vi "demo02_test.vi"() -> ()   [LabVIEW 2017]
panel:
  out "字符串长度":dbl
  in  "字符串":string
  out "数组":dbl[][](array[numeric])
  out "布尔":bool
  out "次数 2":i32
  out "次数":i32
  out "波形图表":dbl(graph)
  out "数值 6":dbl
  in  "数值 5":dbl
  in  "数值 4":dbl
  out "数值 3":dbl
  in  "数值 2":dbl
  in  "数值":dbl
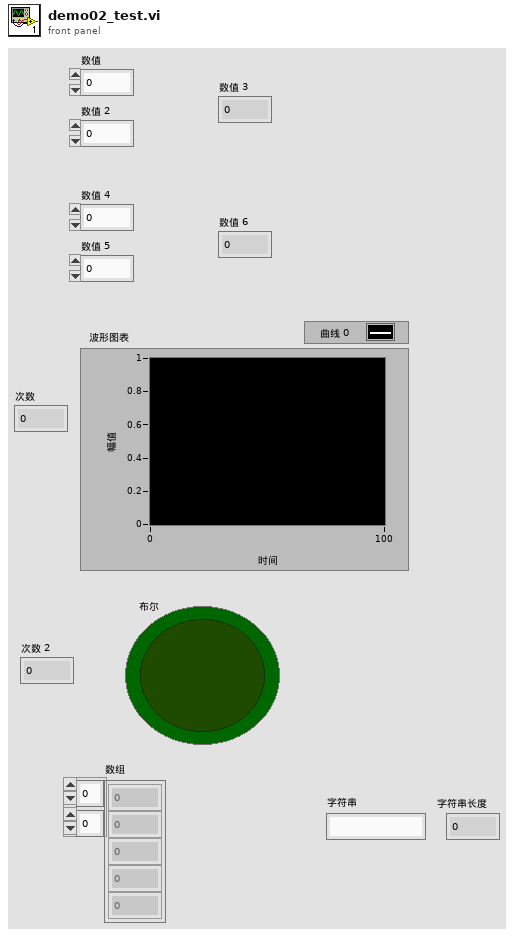
[diagram p1: front panel]
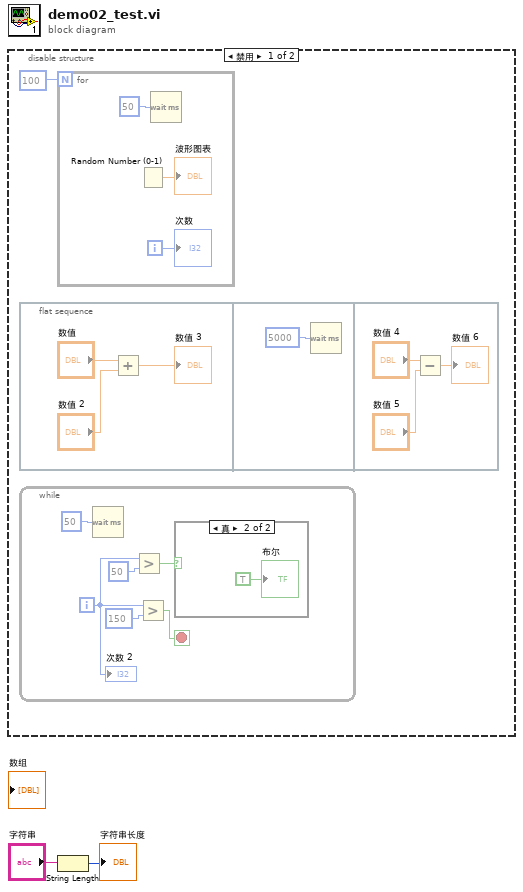
[diagram p0: block diagram]
diagram:
  n1 = disable-structure shown="禁用" {
    frame Disabled {
      n2 = flat-sequence {
        frame #0 {
          n3 = Add(x="数值", y="数值 2") -> (x+y=→"数值 3":dbl)
        }
        frame #1 {
          n4 = Wait (ms)(milliseconds to wait=5000) -> ()  [unwired: 1 out]
        }
        frame #2 {
          n5 = Subtract(x="数值 4", y="数值 5") -> (x-y=→"数值 6":dbl)
        }
      }
      n6 = while {
        i -> [w6]
        stop <- w4 stop-if-true
        n7 = Wait (ms)(milliseconds to wait=u32 50 ("等待时间（毫秒）")) -> ()  [unwired: 1 out]
        n8 = Greater?(x=w6, y=50) -> (0:w7:bool)
        n9 = Greater?(x=w6, y=150) -> (0:w4:bool)
        n10 = case shown="真" w7 {
          frame False {
          }
          frame True {
            "布尔" <- TRUE
          }
        }
        "次数 2" <- w6
      }
      n11 = for {
        N: 100 -> [_]
        i -> [w12]
        n12 = Random Number (0-1)() -> (number: 0 to 1=→"波形图表":dbl)
        n13 = Wait (ms)(milliseconds to wait=u32 50 ("等待时间（毫秒）")) -> ()  [unwired: 1 out]
        "次数" <- w12
      }
    }
    frame Enabled {
    }
  }
  n14 = String Length(string="字符串") -> (length=→"字符串长度":i32)
